vi "position3.vi"() -> ()   [LabVIEW 2023]
panel:
  out "position3":dbl[][](array[numeric])
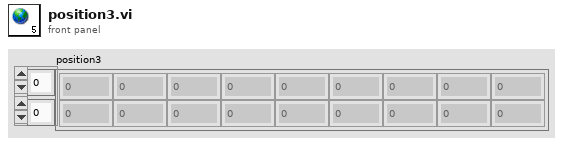
[diagram p1: front panel]
diagram:
